vi "TPNT_WriteTextLog.vi"(6 "UTC":bool, 8 "error in (no error)":errorcluster, 9 "time format":string="%Y-%m-%dT%H:%M:%S", 10 "message":string, 11 "File":path) -> (0 "error out":errorcluster)   [LabVIEW 2016]
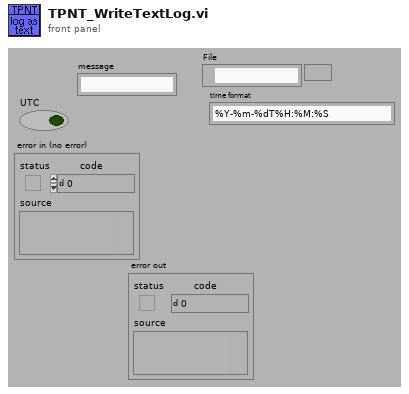
[diagram p1: front panel]
types:
  T1 = enum16{"open", "replace", "create", "open or create", "replace or create", "replace or create with confirmation"}
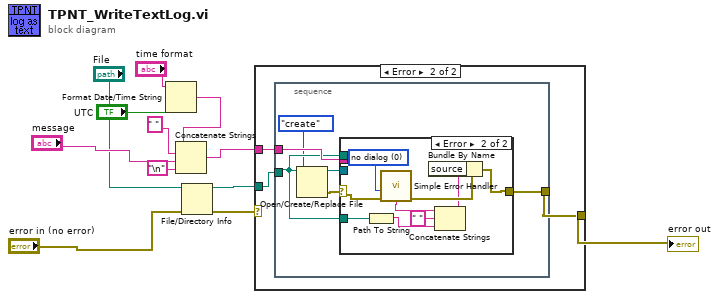
[diagram p0: block diagram]
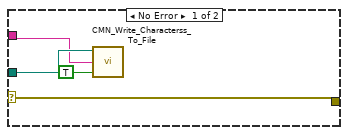
[diagram p2: hidden frame]
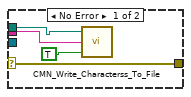
[diagram p3: hidden frame]
diagram:
  n1 = Format Date/Time String(time format string (%c)="time format", UTC format="UTC") -> (date/time string=w8:string)  [unwired: 1 out]
  n2 = Concatenate Strings(w8, " ", "message", "\n") -> (w10:string)
  n3 = File/Directory Info(path="File", error in="error in (no error)") -> (path out=w11:path, error out=w6:errorcluster)  [unwired: 5 out]
  n4 = case shown="Error" w6 {
    selector: w6 -> [w13 _]
    tunnel: w11 -> [w16 w19]
    tunnel: w10 -> [w15 w18]
    tunnel: [w13 w17] -> w2
    frame No Error {
      n5 = call "CMN_Write_Characterss_To_File.vi"("append to file? (new file:F)"=TRUE, "character string"=w15, "file path (dialog if empty)"=w16) -> ()  [unwired: 3 out]
    }
    frame Error {
      n6 = stacked-sequence {
        tunnel: w19 -> [w21]
        tunnel: w18 -> [w24]
        tunnel: [w22] -> w17
        frame #0 {
          n7 = Open/Create/Replace File(file path (use dialog)=w21, operation (0:open)=T1."create") -> (refnum out=w23:refnum<file>, error out=w25:errorcluster)  [unwired: 1 in, 4 out]
          n8 = case shown="Error" w25 {
            selector: w25 -> [w26 w38]
            tunnel: w24 -> [w28 _]
            tunnel: w23 -> [_ _]
            tunnel: w21 -> [w27 _]
            tunnel: [w26 w35] -> w22
            tunnel: w21 -> [_ w33]
            frame No Error {
              n9 = call "CMN_Write_Characterss_To_File.vi"("append to file? (new file:F)"=TRUE, "character string"=w28, "file path (dialog if empty)"=w27) -> ()  [unwired: 3 out]
            }
            frame Error {
              w37 = u16 0 items=["no dialog", "OK message", "continue or stop message"] ("type of dialog (OK msg:1)")
              n10 = Path To String(path=w33) -> (string=w32:string)
              n11 = call <vilib>:"Simple Error Handler.vi"("type of dialog (OK msg:1)"=w37, "error in (no error)"=w38) -> ("error out"=w36:errorcluster, "message"=w34:string)  [unwired: 6 out]
              n12 = Concatenate Strings(w34, " " ("string"), w32) -> (w30:string)
              n13 = Bundle By Name(cluster=w36, "source"=w30) -> (w35:errorcluster)
            }
          }
        }
      }
    }
  }
  "error out" <- w2
